vi "2_3_Causal delay system.vi"(2 "DELAY":i32(knob)=10 scale=-10.0..100.0, 4 "Pulse width":i32=6, 5 "Pulse delay":i32=1, 6 "duty cycle (%)":dbl=50.0 format="%0.2f", 7 "reset phase":bool=TRUE, 8 "samples":i32=100, 9 "Frequency":dbl=80.0 format="%#_6p", 10 "Amplitude":dbl=1.0, 11 "Signal Type":T1(ring)=enum."Pulse") -> (0 "?":dbl[](graph)=[-1.5612511283791264e-17, 4.4188861825309594e-17, -7.743516386535595e-18, -1.3877787807814457e-16, -1.7375905177214616e-17, -1.114316722263881e-16, -2.5602417863708482e-17, -4.4433130751472835e-17, -5.166414918690714e-17, 7.340382915699836e-17, -3.019057850907814e-17, 1.0000000000000004, 1.0, 1.0, 1.0, 0.9999999999999998, 1.0, -1.1148194201611086e-16, -3.283660170461953e-17, 4.007146416971184e-17, -8.224677560860887e-18, 8.770200865447682e-17, 2.1008917116680286e-17, 1.2061436093654783e-16, -3.223891901144718e-17, -5.709545835924507e-17, -2.211353441690445e-17, -9.918986809508961e-17, -2.7120025340888157e-17, 5.204926418401939e-17, -1.5327584577863469e-18, 4.185571952397556e-17, 1.2738327320924897e-17, -4.4305377831858535e-17, 1.110142187857915e-17, -2.817649011180188e-17, -2.558013727430557e-17, 7.984870527692123e-18, -3.485634149656703e-17, -7.81728193858879e-18, -7.32481338042979e-18, -3.815028619916841e-18, 1.7234987356086333e-17, -2.830514475074359e-17, -3.6140140836227164e-17, -3.67168856675507e-18, 2.0100203485039448e-17, -2.5148896273530686e-17, -1.5830778563355095e-17, 2.4136219718743994e-18, 1.7685870865825172e-17, -9.687031795691685e-18, -1.9799176598967157e-17, 1.1990854179401466e-17, -3.4170121295674176e-17, 2.078876204397976e-17, 8.224096923014179e-18, 8.619246103452091e-18, 2.1257773586904425e-17, -7.8274008671008e-18, -2.421788622843889e-17, 2.2766290024734845e-18, 1.0846210506449411e-17, 7.010068590456001e-18, -2.949029909160572e-17, -2.259799199979748e-17, -2.7414197482197333e-17, -1.734723475976807e-17, 1.4849390929546673e-17, 1.3136559004136486e-18, -2.039824743577806e-17, 1.450424336847704e-17, -1.741784921157918e-18, 3.970820531930415e-18, -1.915306286122796e-17, 5.767955557622884e-17, 3.355605723842636e-17, 4.3109741850507616e-17, 2.3845671531103063e-17, 1.5603193921371467e-17, 1.5680273919571608e-17, -1.8622508761532455e-17, -1.2830232269400083e-17, -2.7499616785620394e-17, 8.173746555607062e-18, 1.1332584602429105e-17, -1.4542768848835423e-18, 3.4980025052075225e-18, 1.218197906081555e-17, -1.448507681417907e-17, 5.393351258052734e-18, -2.4803691785905656e-17, -1.4025222796806525e-17, -2.9326258164798306e-17, -1.3065219254052696e-17, -2.5580653026363218e-17, -2.483032616147761e-17, -1.2256580649516176e-17, 6.153614865941503e-19, 1.6114404743474637e-18], 1 "?":dbl[](graph)=[0.0, 1.0, 1.0, 1.0, 1.0, 1.0, 1.0, 0.0, 0.0, 0.0, 0.0, 0.0, 0.0, 0.0, 0.0, 0.0, 0.0, 0.0, 0.0, 0.0, 0.0, 0.0, 0.0, 0.0, 0.0, 0.0, 0.0, 0.0, 0.0, 0.0, 0.0, 0.0, 0.0, 0.0, 0.0, 0.0, 0.0, 0.0, 0.0, 0.0, 0.0, 0.0, 0.0, 0.0, 0.0, 0.0, 0.0, 0.0, 0.0, 0.0, 0.0, 0.0, 0.0, 0.0, 0.0, 0.0, 0.0, 0.0, 0.0, 0.0, 0.0, 0.0, 0.0, 0.0, 0.0, 0.0, 0.0, 0.0, 0.0, 0.0, 0.0, 0.0, 0.0, 0.0, 0.0, 0.0, 0.0, 0.0, 0.0, 0.0, 0.0, 0.0, 0.0, 0.0, 0.0, 0.0, 0.0, 0.0, 0.0, 0.0, 0.0, 0.0, 0.0, 0.0, 0.0, 0.0, 0.0, 0.0, 0.0, 0.0], 3 "Message Box":string="The second graph shows the delayed response")   [LabVIEW 2009]
doc: "This VI emulates a causal delay system."
uses:
  <vilib>/Analysis/2dsp.llb/1D Convolution (DBL).vi
  <vilib>/Analysis/NI_AALBase.lvlib
  <vilib>/Analysis/NI_AALPro.lvlib
panel:
  out "?":bool=TRUE
  out "?":bool=TRUE
  in  "stop":bool
  in  "Impulse delay":i32
  # "Program Developed by Indranil Sinharoy"
  # "Causal delay function"
  # "Square wave"
  # "Impulse wave"
  # "Pulse wave"
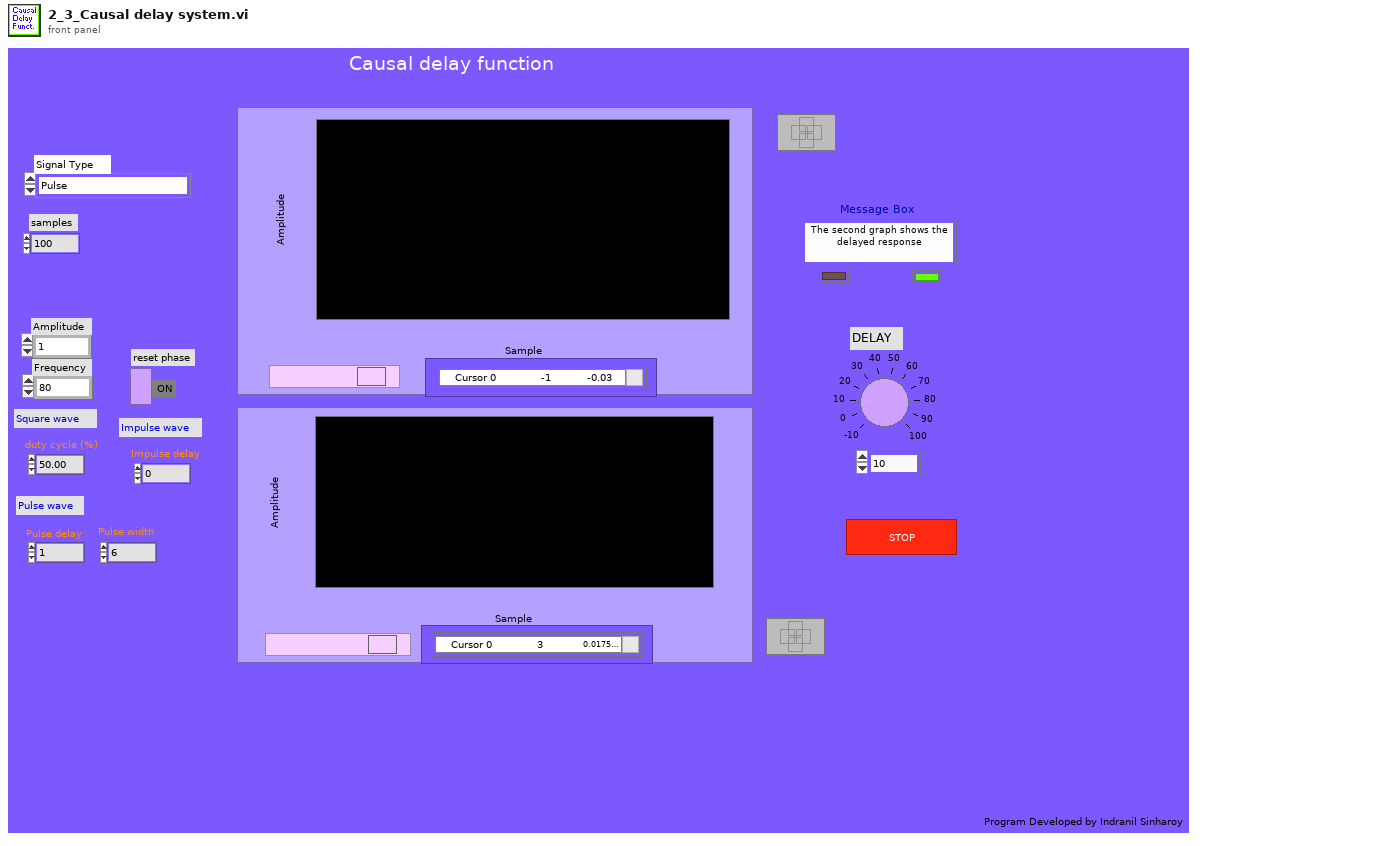
[diagram p1: front panel]
types:
  T1 = enum16{"sine", "square", "Triangular", "Pulse", "Impulse"}
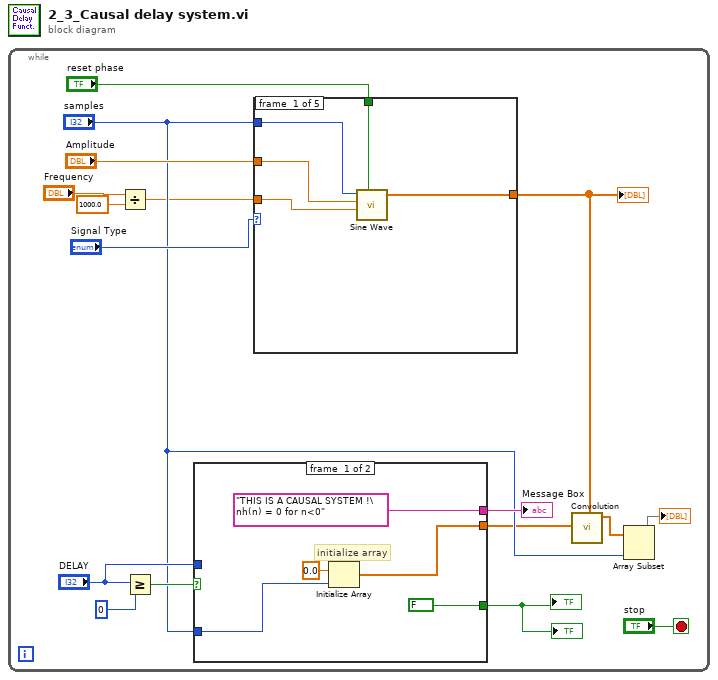
[diagram p0: block diagram]
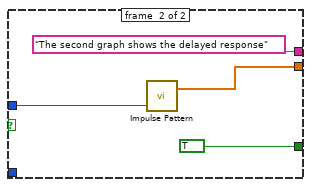
[diagram p2: hidden frame]
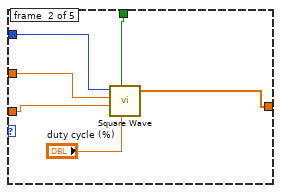
[diagram p3: hidden frame]
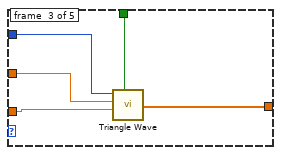
[diagram p4: hidden frame]
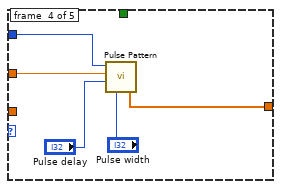
[diagram p5: hidden frame]
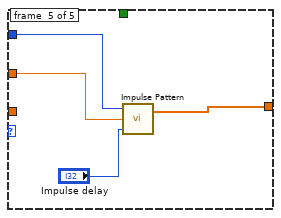
[diagram p6: hidden frame]
diagram:
  n1 = while {
    stop <- "stop" stop-if-true
    n2 = Divide(x="Frequency", y=1000.0) -> (x/y=w3:dbl)
    n3 = Greater Or Equal?(x="DELAY", y=0) -> (x >= y?=w12:bool)
    n4 = case shown="False" w12 {
      tunnel: "DELAY" -> [_ w26]
      tunnel: [w18 w25] -> w6
      tunnel: "samples" -> [w22 _]
      tunnel: [FALSE TRUE] -> w8
      tunnel: ["THIS IS A CAUSAL SYSTEM !\nh(n) = 0 for n<0" ("String") "The second graph shows the delayed response" ("String")] -> w9
      frame #0 {
        # "initialize array"
        n5 = Initialize Array(0.0 ("element"), w22) -> (w18:dbl[])
      }
      frame #1 {
        n6 = call <vilib>:"Impulse Pattern.vi"("delay"=w26) -> ("Impulse Pattern"=w25:dbl[])  [unwired: 2 in, 1 out]
      }
    }
    "?" <- w8
    "Message Box" <- w9
    "?" <- w8
    n7 = case shown="\"Triangular\"" "Signal Type" {
      tunnel: "samples" -> [w31 w36 w41 w47 w51]
      tunnel: "Amplitude" -> [w30 w35 w40 w46 w50]
      tunnel: w3 -> [w29 w34 w39 _ _]
      tunnel: "reset phase" -> [w28 w37 w42 _ _]
      tunnel: [w27 w32 w38 w45 w49] -> w14
      frame #0 {
        n8 = call <vilib>:"Sine Wave.vi"("samples"=w31, "amplitude"=w30, "frequency"=w29, "reset phase"=w28) -> ("sine wave"=w27:dbl[])  [unwired: 1 in, 2 out]
      }
      frame #1 {
        n9 = call <vilib>:"Square Wave.vi"("samples"=w36, "reset phase"=w37, "amplitude"=w35, "frequency"=w34, "duty cycle (%)"="duty cycle (%)") -> ("square wave"=w32:dbl[])  [unwired: 1 in, 2 out]
      }
      frame #2 {
        n10 = call <vilib>:"Triangle Wave.vi"("samples"=w41, "amplitude"=w40, "frequency"=w39, "reset phase"=w42) -> ("triangle wave"=w38:dbl[])  [unwired: 1 in, 2 out]
      }
      frame #3 {
        n11 = call <vilib>:"Pulse Pattern.vi"("width"="Pulse width", "delay"="Pulse delay", "amplitude"=w46, "samples"=w47) -> ("Pulse Pattern"=w45:dbl[])  [unwired: 1 out]
      }
      frame #4 {
        n12 = call <vilib>:"Impulse Pattern.vi"("delay"="Impulse delay", "amplitude"=w50, "samples"=w51) -> ("Impulse Pattern"=w49:dbl[])  [unwired: 1 out]
      }
    }
    "?" <- w14
    n13 = call-poly <vilib>:"Convolution.vi"("Y"=w6, "X"=w14) -> ("X * Y"=w5:dbl[])  [unwired: 8 in, 1 out]
    n14 = Array Subset(array=w5, length="samples") -> (→"?":dbl[])  [unwired: 1 in]
  }
